vi "读取数据文件.vi"(7 "tdms文件路径":path, 8 "错误输入（无错误）":errorcluster) -> (0 "错误输出":errorcluster, 3 "数据":cluster{"扫描":T1[], "脉冲":T1[], "维持时间":T1[]}, 5 "tdms文件输出":refnum<k34>)   [LabVIEW 2021]
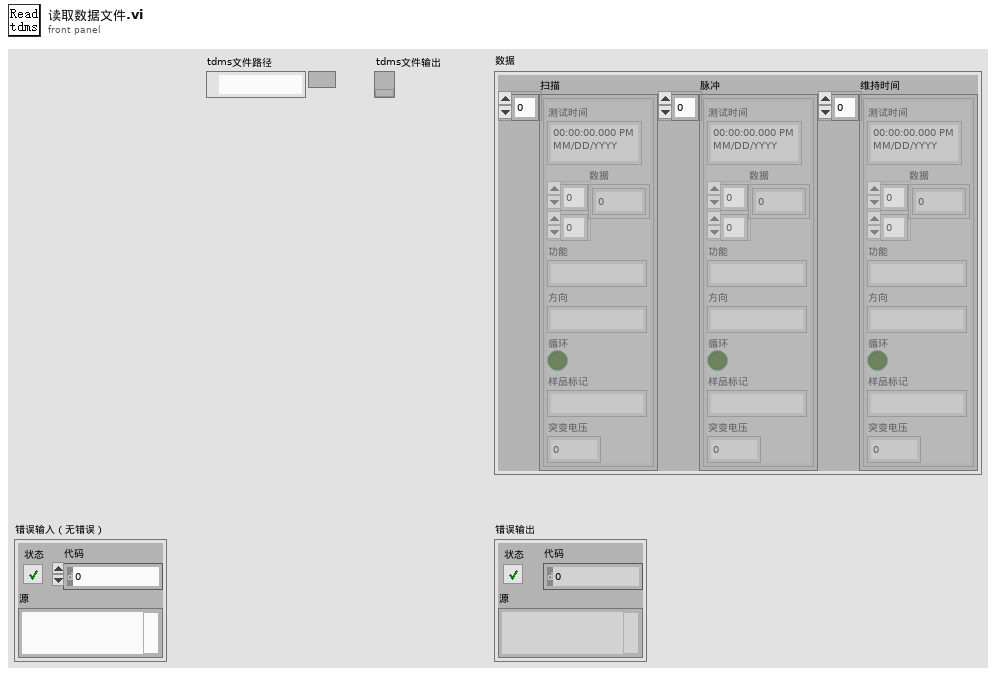
[diagram p1: front panel]
types:
  T1 = typedef "测试数据类型.ctl" = cluster{"测试时间":timestamp, "数据":dbl[][], "功能":string, "方向":string, "循环":bool, "样品标记":string, "突变电压":dbl}
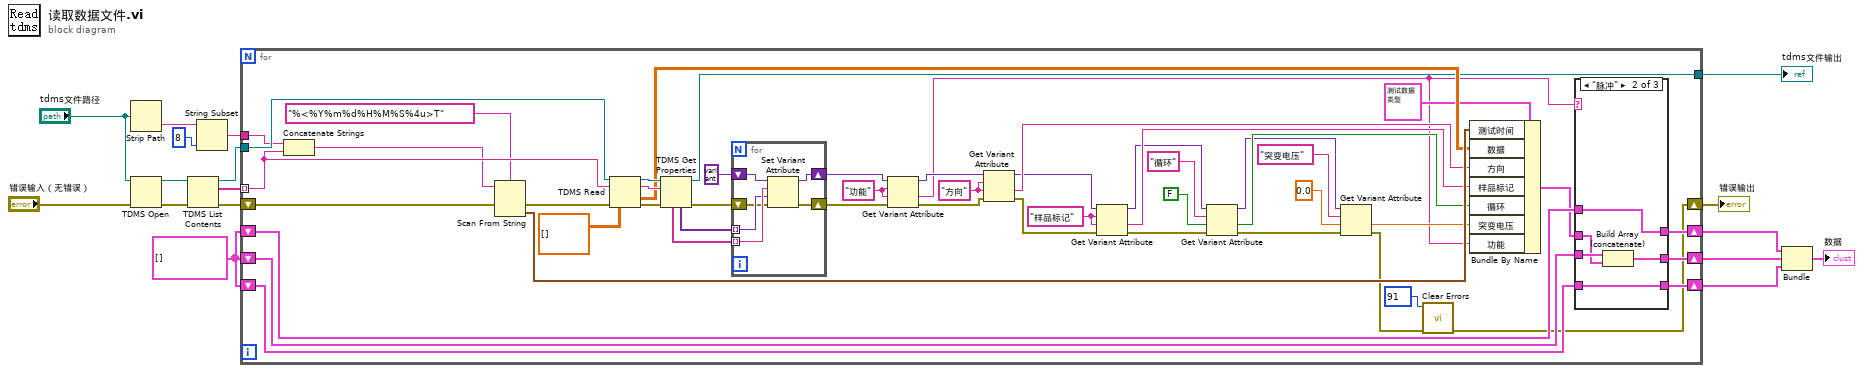
[diagram p0: block diagram]
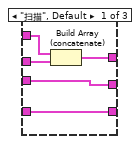
[diagram p2: hidden frame]
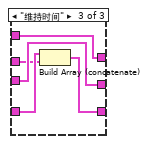
[diagram p3: hidden frame]
diagram:
  w10 = T1[] []
  n1 = Strip Path(path="tdms文件路径") -> (name=w13:string)  [unwired: 1 out]
  n2 = TDMS Open(8:"错误输入（无错误）", 11:"tdms文件路径") -> (0:w8:errorcluster, 3:w17:refnum<k34>)  [unwired: 5 in]
  n3 = TDMS List Contents(4:w8, 7:w17) -> (0:w9:errorcluster, 2:w15:string[], 3:w16:refnum<k34>)  [unwired: 1 in, 1 out]
  n4 = String Subset(string=w13, length (rest)=8 ("长度（剩余）")) -> (substring=w11:string)  [unwired: 1 in]
  n5 = for {
    tunnel: w16 -> [w68]
    tunnel: w15 -> [w67] mode=indexing
    tunnel: w11 -> [w65]
    shift-right: [w52] -> w3
    shift-left: w10 -> [w51]
    shift-right: [w50] -> w2
    shift-left: w10 -> [w49]
    shift-right: [w48] -> w1
    shift-left: w10 -> [w47]
    shift-right: [w19] -> w5
    shift-left: w9 -> [w23]
    tunnel: [w20] -> w6
    w34 = "样品标记" ("名称")
    w33 = "方向" ("名称")
    w56 = "功能" ("名称")
    n6 = Concatenate Strings(w65, w67) -> (w63:string)
    n7 = Scan From String(format string="%<%Y%m%d%H%M%S%4u>T" ("格式字符串"), input string=w63, error in=w23) -> (error out=w22:errorcluster, output 1=w54:timestamp)  [unwired: 2 in, 2 out]
    n8 = TDMS Read(0:w68, 5:w67, 11:w22, 12:dbl[][] []) -> (4:w64:refnum<k34>, 6:w61:string, 10:w53:dbl[][], 15:w31:errorcluster)  [unwired: 4 in, 2 out]
    n9 = TDMS Get Properties(8:w31, 10:w61, 11:w64) -> (0:w30:errorcluster, 3:w20:refnum<k34>, 4:w59:variant[], 6:w60:string[])  [unwired: 3 in, 2 out]
    n10 = for {
      tunnel: w60 -> [w89] mode=indexing
      tunnel: w59 -> [w88] mode=indexing
      shift-right: [w87] -> w57
      shift-left: variant -> [w86]
      shift-right: [w84] -> w29
      shift-left: w30 -> [w85]
      n11 = Set Variant Attribute(Variant=w86, name=w89, value=w88, error in=w85) -> (Variant out=w87:variant, error out=w84:errorcluster)  [unwired: 1 out]
    }
    n12 = Get Variant Attribute(Variant=w57, name=w56, default value (empty Variant)=w56, error in=w29) -> (duplicate Variant=w55:variant, value=w21:string, error out=w28:errorcluster)  [unwired: 1 out]
    n13 = Get Variant Attribute(Variant=w55, name=w33, default value (empty Variant)=w33, error in=w28) -> (duplicate Variant=w40:variant, value=w46:string, error out=w27:errorcluster)  [unwired: 1 out]
    n14 = Get Variant Attribute(Variant=w40, name=w34, default value (empty Variant)=w34, error in=w27) -> (duplicate Variant=w41:variant, value=w43:string, error out=w26:errorcluster)  [unwired: 1 out]
    n15 = Get Variant Attribute(Variant=w41, name="循环" ("名称"), default value (empty Variant)=FALSE, error in=w26) -> (duplicate Variant=w42:variant, value=w44:bool, error out=w25:errorcluster)  [unwired: 1 out]
    n16 = Get Variant Attribute(Variant=w42, name="突变电压" ("名称"), default value (empty Variant)=0.0, error in=w25) -> (value=w45:dbl, error out=w24:errorcluster)  [unwired: 2 out]
    n17 = call <vilib>:"Clear Errors.vi"("error in (no error)"=w24, "specific error code to clear (0: all)"=91) -> ("error out"=w19:errorcluster)  [unwired: 4 in, 1 out]
    n18 = Bundle By Name(cluster=T1 {"测试时间"=timestamp(0 s since 1904-01-01), "数据"=[], "功能"="", "方向"="", "循环"=FALSE, "样品标记"="", "突变电压"=0.0} ("测试数据"), "测试时间"=w54, "数据"=w53, "方向"=w46, "样品标记"=w43, "循环"=w44, "突变电压"=w45, "功能"=w21) -> (w32:T1)
    n19 = case shown="\"脉冲\"" w21 {
      tunnel: [w73 w78 w83] -> w52
      tunnel: w51 -> [w72 w78 w83]
      tunnel: [w71 w77 w80] -> w50
      tunnel: w49 -> [w71 w76 w80]
      tunnel: [w70 w75 w82] -> w48
      tunnel: w47 -> [w70 w75 w81]
      tunnel: w32 -> [w69 w74 w79]
      frame "扫描", Default {
        n20 = Build Array (concatenate)(w72, w69) -> (w73:T1[])
      }
      frame "脉冲" {
        n21 = Build Array (concatenate)(w76, w74) -> (w77:T1[])
      }
      frame "维持时间" {
        n22 = Build Array (concatenate)(w81, w79) -> (w82:T1[])
      }
    }
  }
  "tdms文件输出" <- w6
  "错误输出" <- w5
  n23 = Bundle(w3, w2, w1) -> (→"数据":cluster{T1[], T1[], T1[]})  [unwired: 1 in]
